vi "test_call.vi"() -> (3 "test_result":T1)   [LabVIEW 2015]
uses:
  tester_result.ctl
  result/result.lvclass/result.ctl
  request/request.lvclass/request.ctl
  <vilib>/addons/lv-msgpack/MsgPack Deserializer/Unflatten From MessagePack.vi
  input/input.lvclass
  output/Output.lvclass
  request/request.lvclass
  result/result.lvclass
  result/result_from_call/result_from_call.lvclass
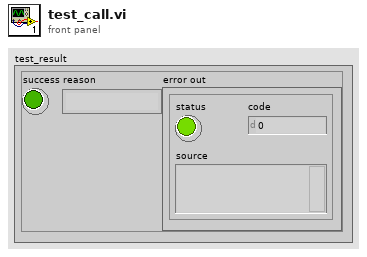
[diagram p1: front panel]
types:
  T1 = typedef "tester_result.ctl" = cluster{"success":bool, "reason":string, "error out":errorcluster}
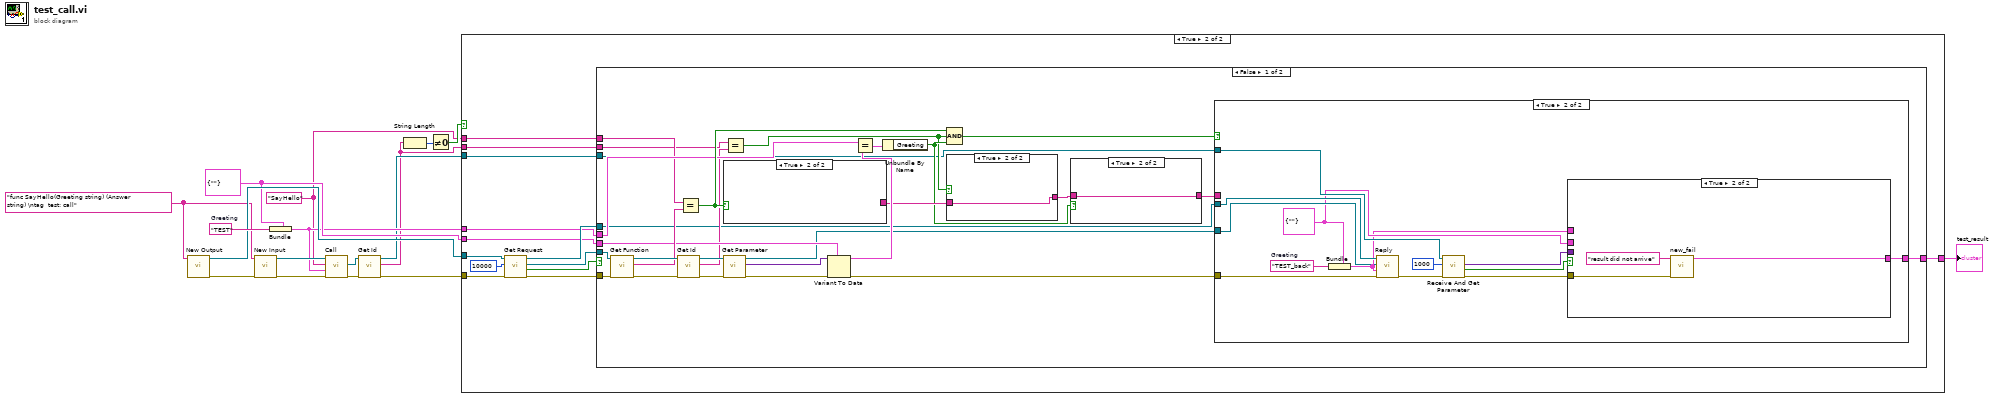
[diagram p0: block diagram]
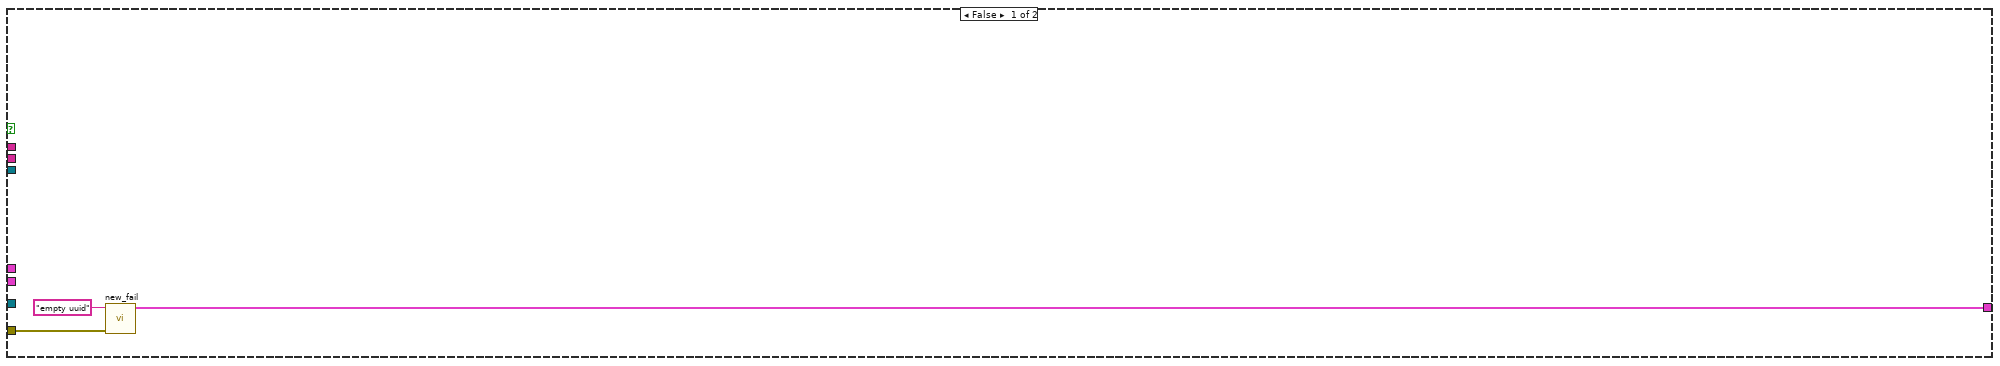
[diagram p2: hidden frame]
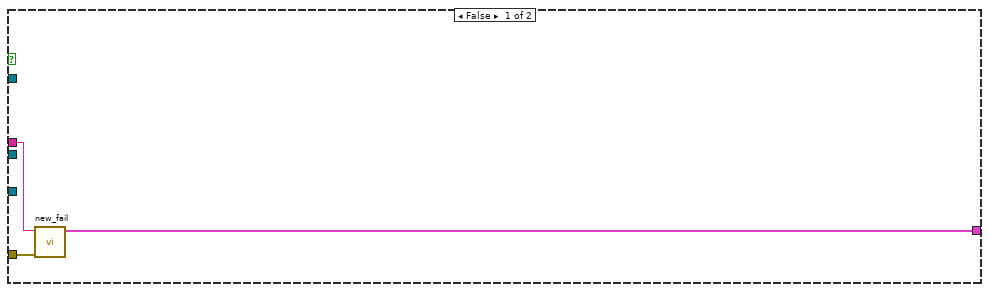
[diagram p3: hidden frame]
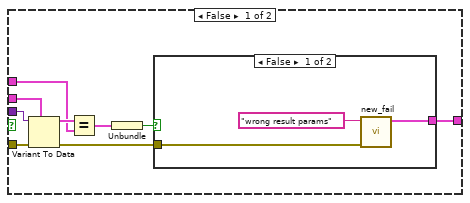
[diagram p4: hidden frame]
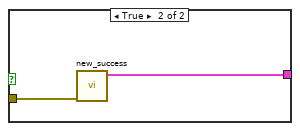
[diagram p5: hidden frame]
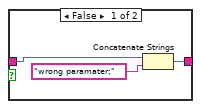
[diagram p6: hidden frame]
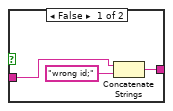
[diagram p7: hidden frame]
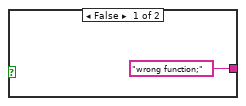
[diagram p8: hidden frame]
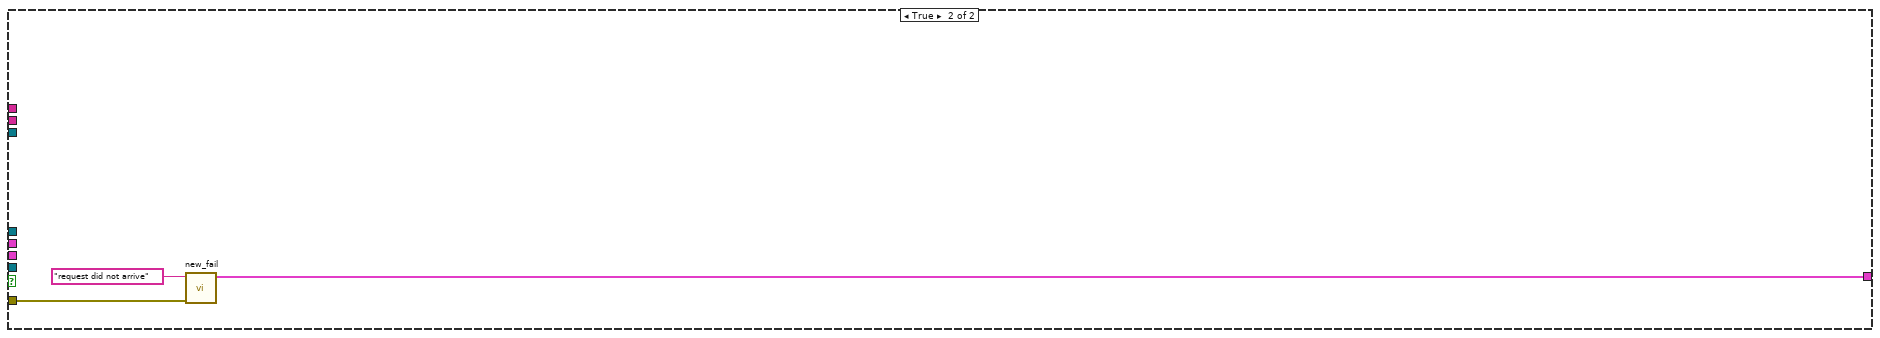
[diagram p9: hidden frame]
diagram:
  w15 = "TEST"  # Greeting
  w8 = cluster{"Greeting":string} {"Greeting"=""}
  w6 = "SayHello" ("Function")
  w9 = "func SayHello(Greeting string) (Answer string) \ntag  test: call" ("Descriptor")
  n1 = call "New Output.vi"("Descriptor"=w9) -> ("error out"=w11:errorcluster, "output"=w10:refnum<class "Output.lvclass">)  [unwired: 9 in]
  n2 = call "New Input.vi"("error in (no error)"=w11, "Descriptor"=w9) -> ("error out"=w16:errorcluster, "input out"=w17:refnum<class "input.lvclass">)  [unwired: 8 in]
  n3 = Bundle(cluster=w8, "Greeting"=w15) -> (w7:cluster{"Greeting":string})
  n4 = call "Call.vi"("error in (no error)"=w16, "Parameter"=w7, "Function"=w6, "input in"=w17) -> ("error out"=w4:errorcluster, "result"=w5:refnum<class "result_from_call.lvclass">)  [unwired: 5 in, 1 out]
  n5 = call "Get Id.vi"("error in (no error)"=w4, "result in"=w5) -> ("error out"=w3:errorcluster, "id"=w1:string, "result out"=w2:refnum<class "result_from_call.lvclass">)  [unwired: 7 in]
  n6 = String Length(string=w1) -> (length=w14:i32)
  n7 = Not Equal To 0?(x=w14) -> (x != 0?=w13:bool)
  n8 = case shown="True" w13 {
    tunnel: w3 -> [w19 w31]
    tunnel: [w18 w28] -> w12
    tunnel: w10 -> [_ w32]
    tunnel: w8 -> [_ w26]
    tunnel: w7 -> [_ w25]
    tunnel: w6 -> [_ w24]
    tunnel: w1 -> [_ w23]
    tunnel: w2 -> [_ w21]
    frame False {
      n9 = call "new_fail.vi"("error out"=w19, "reason"="empty uuid" ("Function")) -> ("result"=w18:T1)  [unwired: 9 in]
    }
    frame True {
      n10 = call "Get Request.vi"("error in (no error)"=w31, "timeout in ms (-1)"=10000, "output in"=w32) -> ("error out"=w29:errorcluster, "timed out?"=w30:bool, "request.lvclass"=w22:refnum<class "request.lvclass">, "output out"=w27:refnum<class "Output.lvclass">)  [unwired: 5 in]
      n11 = case shown="False" w30 {
        tunnel: w29 -> [w38 w105]
        tunnel: [w39 w104] -> w28
        tunnel: w27 -> [w36 _]
        tunnel: w26 -> [w48 _]
        tunnel: w25 -> [w47 _]
        tunnel: w24 -> [w46 _]
        tunnel: w23 -> [w44 _]
        tunnel: w22 -> [w37 _]
        tunnel: w21 -> [w34 _]
        frame False {
          n12 = call "Get Function.vi"("error in (no error)"=w38, "request in"=w37) -> ("error out"=w61:errorcluster, "function"=w57:string, "request out"=w59:refnum<class "request.lvclass">)  [unwired: 7 in]
          n13 = call "Get Id.vi"("error in (no error)"=w61, "request in"=w59) -> ("error out"=w60:errorcluster, "id"=w43:string, "request out"=w58:refnum<class "request.lvclass">)  [unwired: 7 in]
          n14 = Equal?(x=w46, y=w57) -> (x = y?=w50:bool)
          n15 = case shown="True" w50 {
            tunnel: ["wrong function;" ("source") _] -> w53
            frame False {
            }
            frame True {
            }
          }
          n16 = call "Get Parameter.vi"("error in (no error)"=w60, "request in"=w58) -> ("error out"=w56:errorcluster, "parameter"=w55:variant, "request out"=w35:refnum<class "request.lvclass">)  [unwired: 7 in]
          n17 = Equal?(x=w44, y=w43) -> (x = y?=w45:bool)
          n18 = Variant To Data(error in=w56, type=w48, Variant=w55) -> (data=w54:cluster{"Greeting":string}, error out=w41:errorcluster)
          n19 = Equal?(x=w47, y=w54) -> (x = y?=w51:cluster{"Greeting":bool})
          n20 = Unbundle By Name(w51) -> ("Greeting"=w49:bool)
          n21 = Compound Arithmetic op=AND(w50, w45, w49) -> (w40:bool)
          n22 = case shown="True" w45 {
            tunnel: w53 -> [w101 w102]
            tunnel: [w99 w102] -> w52
            frame False {
              n23 = Concatenate Strings(w101, "wrong id;" ("source")) -> (w99:string)
            }
            frame True {
            }
          }
          n24 = case shown="True" w49 {
            tunnel: w52 -> [w97 w98]
            tunnel: [w95 w98] -> w42
            frame False {
              n25 = Concatenate Strings(w97, "wrong paramater;" ("source")) -> (w95:string)
            }
            frame True {
            }
          }
          n26 = case shown="True" w40 {
            tunnel: w42 -> [w64 _]
            tunnel: w41 -> [w63 w76]
            tunnel: [w62 w65] -> w39
            tunnel: w36 -> [_ w75]
            tunnel: w35 -> [_ w74]
            tunnel: w34 -> [_ w72]
            frame False {
              n27 = call "new_fail.vi"("error out"=w63, "reason"=w64) -> ("result"=w62:T1)  [unwired: 9 in]
            }
            frame True {
              w77 = "TEST_back"  # Greeting
              w67 = cluster{"Answer":string} {"Answer"=""}
              n28 = Bundle(cluster=w67, "Answer"=w77) -> (w66:cluster{"Answer":string})
              n29 = call "Reply.vi"("error in (no error)"=w76, "parameter"=w66, "request"=w74, "output in"=w75) -> ("error out"=w71:errorcluster)  [unwired: 6 in, 1 out]
              n30 = call "Receive And Get Parameter.vi"("error in (no error)"=w71, "timeout in ms (-1)"=1000, "result_from_call in"=w72) -> ("error out"=w69:errorcluster, "timeout"=w70:bool, "Data"=w68:variant)  [unwired: 5 in, 1 out]
              n31 = case shown="True" w70 {
                tunnel: w69 -> [w86 w93]
                tunnel: w68 -> [w85 _]
                tunnel: w67 -> [w84 _]
                tunnel: w66 -> [w82 _]
                tunnel: [w78 w92] -> w65
                frame False {
                  n32 = Variant To Data(error in=w86, type=w84, Variant=w85) -> (data=w83:cluster{"Answer":string}, error out=w79:errorcluster)
                  n33 = Equal?(x=w83, y=w82) -> (x = y?=w81:cluster{"Answer":bool})
                  n34 = Unbundle(w81) -> ("Answer"=w80:bool)
                  n35 = case shown="False" w80 {
                    tunnel: w79 -> [w88 w91]
                    tunnel: [w87 w90] -> w78
                    frame False {
                      n36 = call "new_fail.vi"("error out"=w88, "reason"="wrong result params") -> ("result"=w87:T1)  [unwired: 9 in]
                    }
                    frame True {
                      n37 = call "new_success.vi"("error out"=w91) -> ("result"=w90:T1)  [unwired: 10 in]
                    }
                  }
                }
                frame True {
                  n38 = call "new_fail.vi"("error out"=w93, "reason"="result did not arrive") -> ("result"=w92:T1)  [unwired: 9 in]
                }
              }
            }
          }
        }
        frame True {
          n39 = call "new_fail.vi"("error out"=w105, "reason"="request did not arrive" ("Function")) -> ("result"=w104:T1)  [unwired: 9 in]
        }
      }
    }
  }
  "test_result" <- w12
